vi "Information.vi"(8 "error in (no error)":errorcluster, 9 "Context":T1, 10 "Information":refnum<class "Information.lvclass">, 11 "Process Object in":refnum<class "Process Object.lvclass">) -> (0 "error out":errorcluster, 3 "Process Object out":refnum<class "Process Object.lvclass">)   [LabVIEW 2021, in "Process Object.lvclass"]
uses:
  Publish-Subscribe/Interfaces/Information/Information.lvclass
  Publish-Subscribe/Context.ctl
  Process Object.lvclass
  Process Object.lvclass/Process Object.ctl
  NHMFL_Core/Libraries/Instruments/Results/Acquired Result/Acquired Result.lvclass
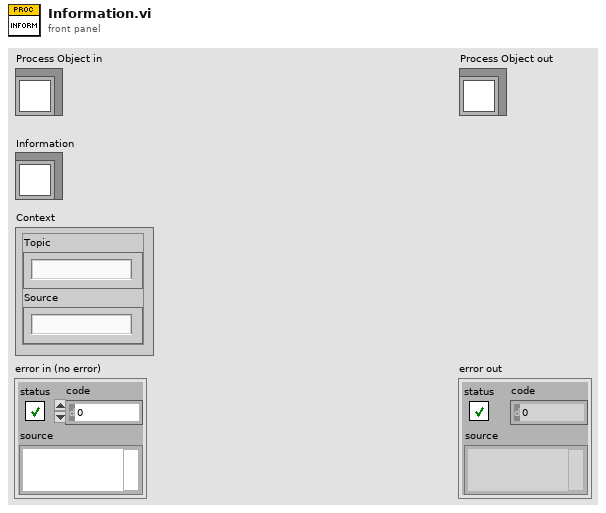
[diagram p1: front panel]
types:
  T1 = typedef "Context.ctl" = cluster{"Topic":string, "Source":string}
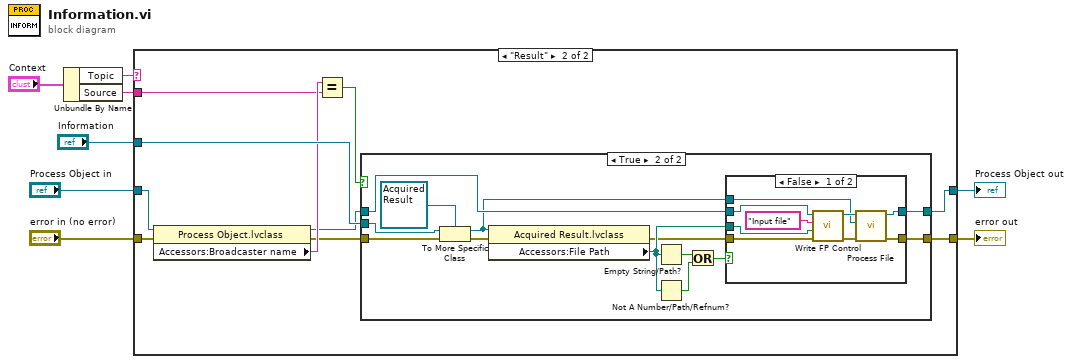
[diagram p0: block diagram]
diagram:
  n1 = Unbundle By Name("Context") -> ("Topic"=w8:string, "Source"=w7:string)
  n2 = case shown="\"Result\"" w8 {
    tunnel: "Information" -> [_ w20]
    tunnel: "error in (no error)" -> [w9 w16]
    tunnel: "Process Object in" -> [w10 w15]
    tunnel: [w10 w19] -> w1
    tunnel: [w9 w18] -> w2
    tunnel: w7 -> [_ w14]
    frame "", Default {
    }
    frame "Result" {
      n3 = property class="Process Object.lvclass"(reference=w15, error in=w16) -> (reference out=w12:refnum<class "Process Object.lvclass">, error out=w11:errorcluster, "Accessors:Broadcaster name"=w17:string)
      n4 = Equal?(x=w17, y=w14) -> (x = y?=w13:bool)
      n5 = case shown="True" w13 {
        tunnel: w20 -> [_ w34]
        tunnel: [w22 w26] -> w19
        tunnel: [w21 w23] -> w18
        tunnel: w11 -> [w21 w33]
        tunnel: w12 -> [w22 w32]
        frame False {
        }
        frame True {
          n6 = To More Specific Class(target class=refnum<class "Acquired Result.lvclass"> refnum ("Acquired Result.lvclass"), reference=w34, error in=w33) -> (specific class reference=w25:refnum<class "Acquired Result.lvclass">, error out=w24:errorcluster)
          n7 = property class="Acquired Result.lvclass"(reference=w25, error in=w24) -> (error out=w27:errorcluster, "Accessors:File Path"=w31:path)  [unwired: 1 out]
          n8 = Empty String/Path?(string/path=w31) -> (empty?=w28:bool)
          n9 = Not A Number/Path/Refnum?(number/path/refnum=w31) -> (NaN/Path/Refnum?=w29:bool)
          n10 = Or(x=w28, y=w29) -> (x .or. y?=w30:bool)
          n11 = case shown="False" w30 {
            tunnel: w32 -> [w40 w46]
            tunnel: w27 -> [w44 w45]
            tunnel: [w38 w46] -> w26
            tunnel: [w37 w45] -> w23
            tunnel: w25 -> [w39 _]
            tunnel: w31 -> [w36 _]
            frame False {
              n12 = call-dynamic "Write FP Control.vi"("error in (no error)"=w44, "Control Value"=w36, "Control Name"="Input file", "Measure Object in"=w40) -> ("error out"=w42:errorcluster, "Measure Object out"=w41:refnum<class "Process Object.lvclass">)  [unwired: 6 in]
              n13 = call-dynamic "Process File.vi"("error in (no error)"=w42, "Result in"=w39, "Process Object in"=w41) -> ("error out"=w37:errorcluster, "Process Object out"=w38:refnum<class "Process Object.lvclass">)  [unwired: 6 in, 1 out]
            }
            frame True {
            }
          }
        }
      }
    }
  }
  "error out" <- w2
  "Process Object out" <- w1
